vi "WheelShoot.vi"(8 "error in (no error)":errorcluster, 10 "Power":dbl) -> (0 "error out":errorcluster)   [LabVIEW 2015]
doc: "Spins up the firing motors and then shoots over one second."
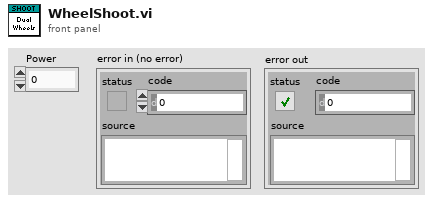
[diagram p1: front panel]
types:
  T1 = typedef "WPI_ServoDeviceRef.ctl" = cluster{"DeviceStatus":errorcluster, "PWM Channel":T2, "DeadBand":T3}
  T2 = typedef "FPGA_DIOPWMChannel.ctl" = enum8{"PWM 0", "PWM 1", "PWM 2", "PWM 3", "PWM 4", "PWM 5", "PWM 6", "PWM 7", "PWM 8", "PWM 9", "PWM MXP 0", "PWM MXP 1", "PWM MXP 2", "PWM MXP 3", "PWM MXP 4", "PWM MXP 5", "PWM MXP 6", "PWM MXP 7", "PWM MXP 8", "PWM MXP 9", "Invalid"}
  T3 = typedef "WPI_PWMDeadband.ctl" = cluster{"Name":string, "maxPositivePwm":i32, "minPositivePwm":i32, "centerPwm":i32, "maxNegativePwm":i32, "minNegativePwm":i32, "angularRange":u16}
  T4 = typedef "WPI_MotorControlDeviceRef.ctl" = cluster{"DeviceStatus":errorcluster, "Type":T5, "PWM":cluster{"PWM Channel":T2, "DeadBand":T3}, "CAN":cluster{"Device Number":u8, "Control Mode":T6, "Semaphore":T7, "Max Vout":dbl, "TalonSRX Control Mode":T8}, "Invert":bool}
  T5 = typedef "WPI_MotorControlType.ctl" = enum16{"PWM", "CAN", "CANTalonSRX"}
  T6 = typedef "WPI_CANJaguar_ControlMode.ctl" = enum8{"Percent VBus", "Current", "Speed", "Position", "Voltage"}
  T7 = typedef "Semaphore RefNum" = refnum<k1>
  T8 = typedef "WPI_CANTalonSRX_APIControlMode.ctl" = enum8{"Percent VBus", "Speed", "Position", "Slave", "Unchanged / Invalid", "Voltage Compensation", "Current", "Motion Profile"}
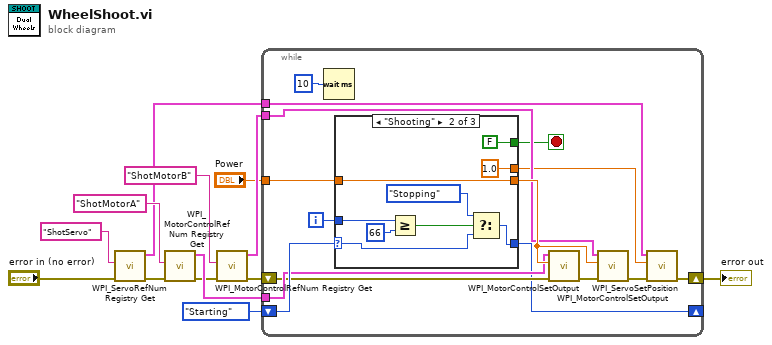
[diagram p0: block diagram]
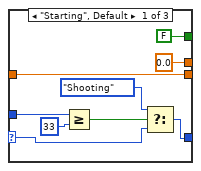
[diagram p2: hidden frame]
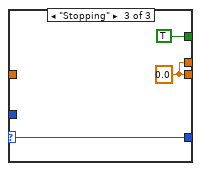
[diagram p3: hidden frame]
diagram:
  n1 = call <vilib>:"WPI_ServoRefNum Registry Get.vi"("error in (no error)"="error in (no error)", "refnum name"="ShotServo") -> ("error out"=w2:errorcluster, "ServoDeviceRef"=w1:T1)  [unwired: 8 in]
  n2 = call <vilib>:"WPI_MotorControlRefNum Registry Get.vi"("error in (no error)"=w2, "refnum name"="ShotMotorA") -> ("error out"=w8:errorcluster, "MotorControlDevRef"=w10:T4)  [unwired: 8 in]
  n3 = call <vilib>:"WPI_MotorControlRefNum Registry Get.vi"("error in (no error)"=w8, "refnum name"="ShotMotorB") -> ("error out"=w7:errorcluster, "MotorControlDevRef"=w11:T4)  [unwired: 8 in]
  n4 = while {
    shift-right: [w18] -> _
    shift-left: enum16{"Starting", "Shooting", "Stopping"}."Starting" -> [w28]
    tunnel: "Power" -> [w27]
    tunnel: w10 -> [w25]
    tunnel: w11 -> [w24]
    shift-right: [w15] -> w6
    shift-left: w7 -> [w20]
    tunnel: w1 -> [w17]
    i -> [w23]
    stop <- w21 stop-if-true
    n5 = Wait (ms)(milliseconds to wait=u32 10) -> ()  [unwired: 1 out]
    n6 = case shown="\"Shooting\"" w28 {
      selector: w28 -> [w34 w40 w49]
      tunnel: [w33 w45 w49] -> w18
      tunnel: [w31 w46 w47] -> w26
      tunnel: w27 -> [w31 w46 _]
      tunnel: w23 -> [w36 w43 _]
      tunnel: [FALSE FALSE TRUE] -> w21
      tunnel: [0.0 1.0 w47] -> w14
      frame "Starting", Default {
        n7 = Greater Or Equal?(x=w36, y=33) -> (x >= y?=w37:bool)
        n8 = Select(t=enum16{"Starting", "Shooting", "Stopping"}."Shooting", s=w37, f=w34) -> (s? t:f=w33:enum16{"Starting", "Shooting", "Stopping"})
      }
      frame "Shooting" {
        n9 = Greater Or Equal?(x=w43, y=66) -> (x >= y?=w44:bool)
        n10 = Select(t=enum16{"Starting", "Shooting", "Stopping"}."Stopping", s=w44, f=w40) -> (s? t:f=w45:enum16{"Starting", "Shooting", "Stopping"})
      }
      frame "Stopping" {
        w47 = 0.0 ("Power")
      }
    }
    n11 = call <vilib>:"WPI_MotorControlSetOutput.vi"("error in (no error)"=w20, "Output"=w26, "MotorControlDevRef"=w25) -> ("error out"=w19:errorcluster)  [unwired: 6 in, 2 out]
    n12 = call <vilib>:"WPI_MotorControlSetOutput.vi"("error in (no error)"=w19, "Output"=w26, "MotorControlDevRef"=w24) -> ("error out"=w16:errorcluster)  [unwired: 6 in, 2 out]
    n13 = call <vilib>:"WPI_ServoSetPosition.vi"("error in (no error)"=w16, "Position"=w14, "ServoDeviceRef"=w17) -> ("error out"=w15:errorcluster)  [unwired: 7 in, 1 out]
  }
  "error out" <- w6
